vi "PanelUpdates_Defer.vi"(8 "error in (no error)":errorcluster, 11 "Parent VI Reference":refnum<vi>) -> (0 "error out":errorcluster)   [LabVIEW 2020, in "hse-ui.lvlib"]
doc: "____\nHAMPEL SOFTWARE ENGINEERING v3.8.0 (2023-12-18 14:41)"
uses:
  hse-ui.lvlib
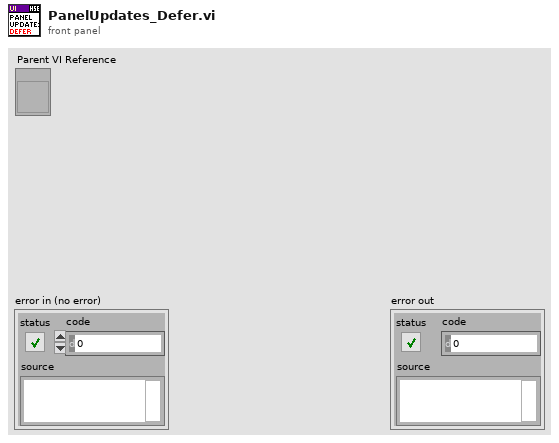
[diagram p1: front panel]
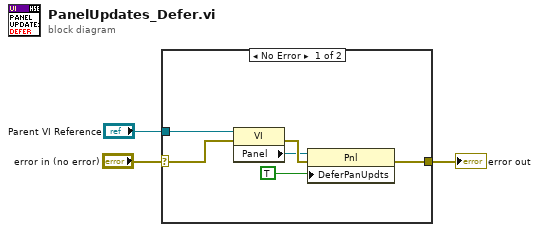
[diagram p0: block diagram]
diagram:
  n1 = case shown="No Error" "error in (no error)" {
    selector: "error in (no error)" -> [w5 w10]
    tunnel: "Parent VI Reference" -> [w8 _]
    tunnel: [w4 w10] -> w1
    frame No Error {
      n2 = property class="VI"(reference=w8, error in=w5) -> (error out=w7:errorcluster, "Panel"=w6:refnum<vi>)  [unwired: 1 out]
      n3 = property class="Pnl"(reference=w6, error in=w7, "DeferPanUpdts"=TRUE ("Defer Panel Updates")) -> (error out=w4:errorcluster)  [unwired: 1 out]
    }
    frame Error {
    }
  }
  "error out" <- w1
